vi "GetMethodImage.vi"(8 "error in (no error)":errorcluster, 9 "MethodVI":path, 10 "MethodName":string) -> (0 "error out":errorcluster, 2 "MethodImage":T2)   [LabVIEW 2020, in "ClassWriterNative.lvclass"]
uses:
  ClassWriterNative.lvclass
  <vilib>/picture/picture.llb/imagedata.ctl
  <vilib>/Utility/config.llb/Read Key (String).vi
  <vilib>/regexp/Match Regular Expression.xnode
  ClassWriterNative.lvclass/ClassWriterNative.ctl
  <vilib>/Utility/config.llb/NI_LVConfig.lvlib
panel:
  out "2D Picture":picture
  out "Array":T1(array[cluster])
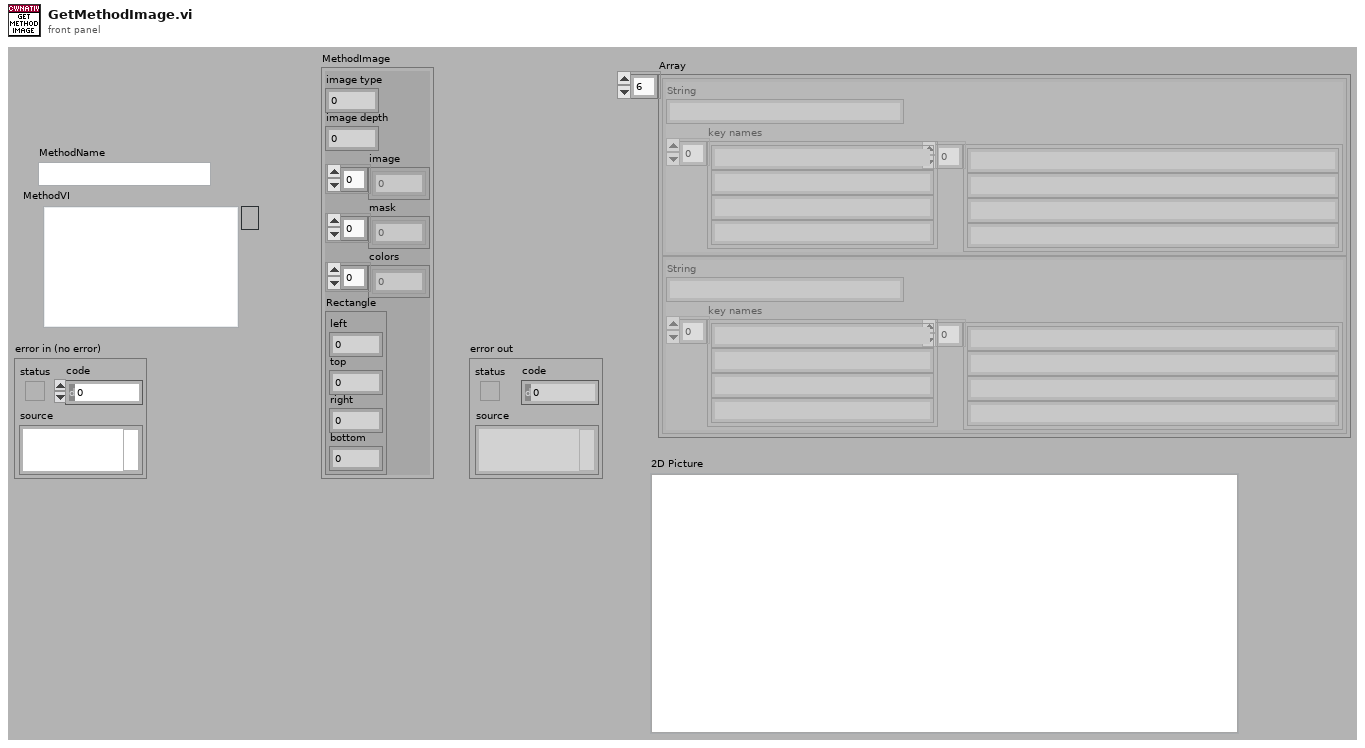
[diagram p1: front panel]
types:
  T1 = cluster{"String":string, "key names":string[], string[]}[]
  T2 = typedef "imagedata.ctl" = cluster{"image type":i32, "image depth":i32, "image":u8[], "mask":u8[], "colors":u32[], "Rectangle":cluster{"left":i16, "top":i16, "right":i16, "bottom":i16}}
  T3 = cluster{string, "key names":string[], string[]}[]
  T4 = typedef "NI_LVConfig.lvlib/Config Data RefNum.ctl" = refnum<k1>
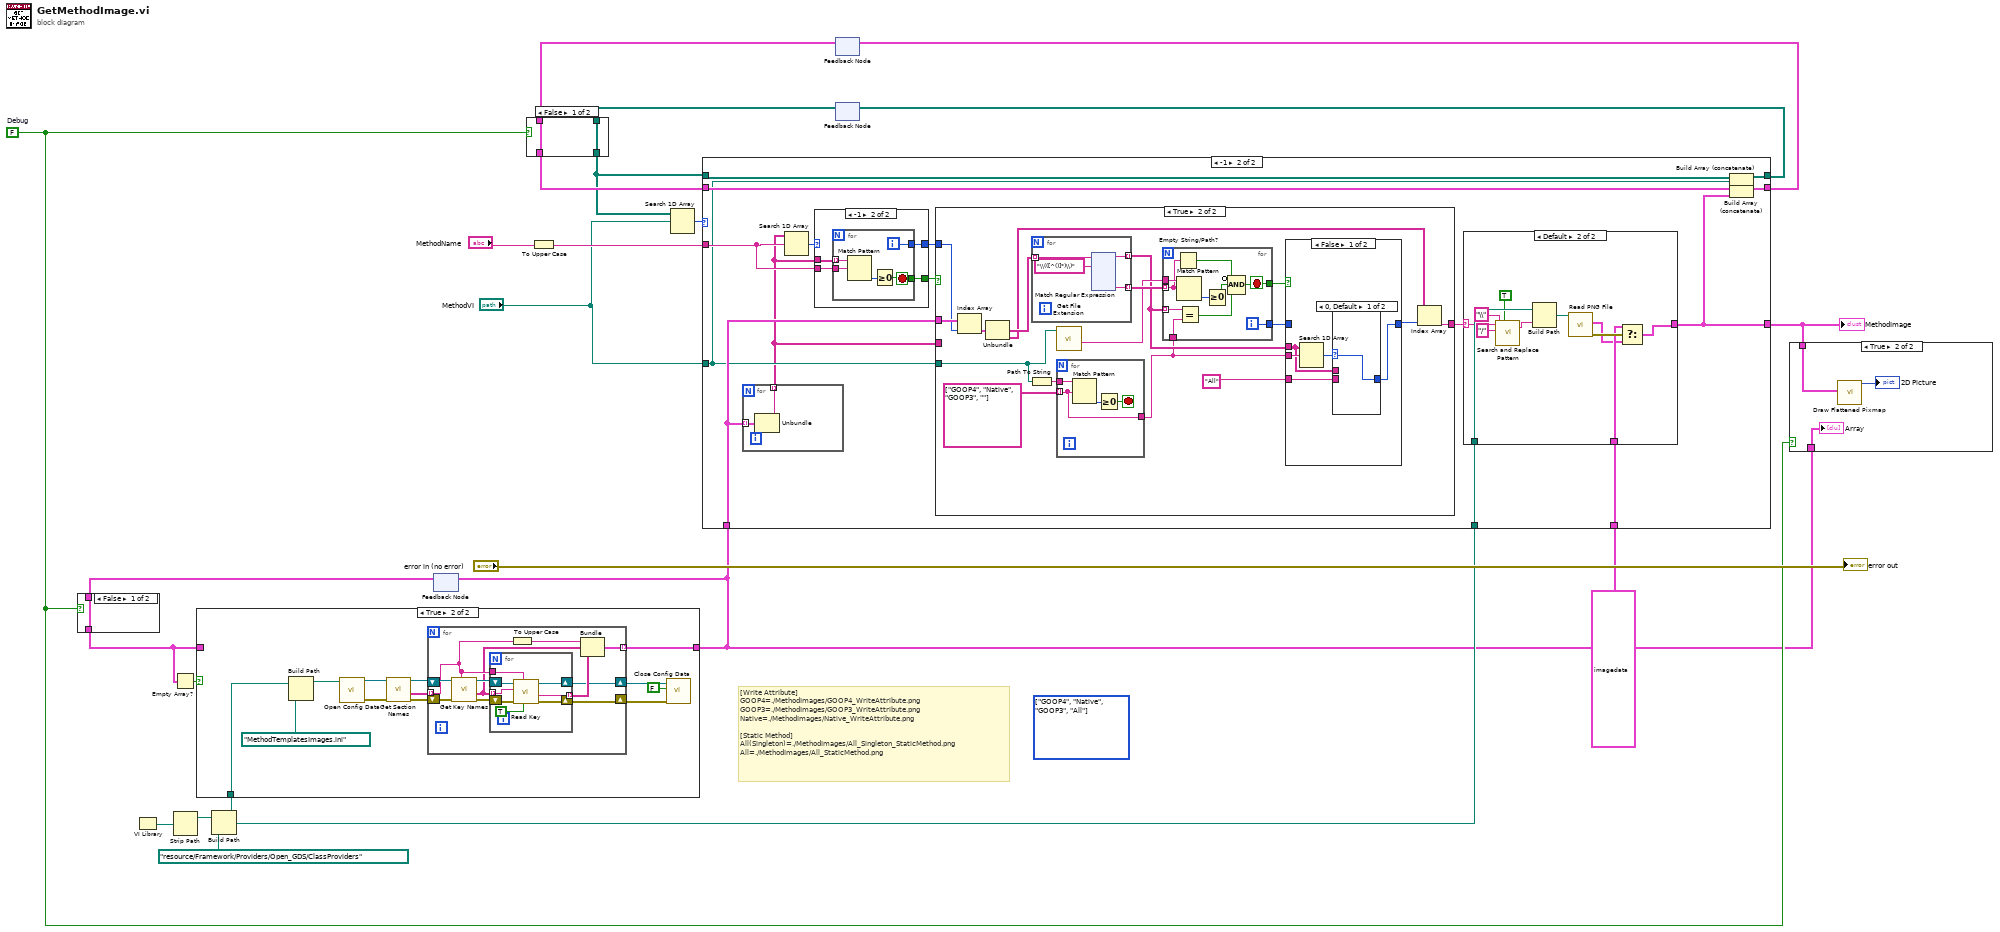
[diagram p0: block diagram]
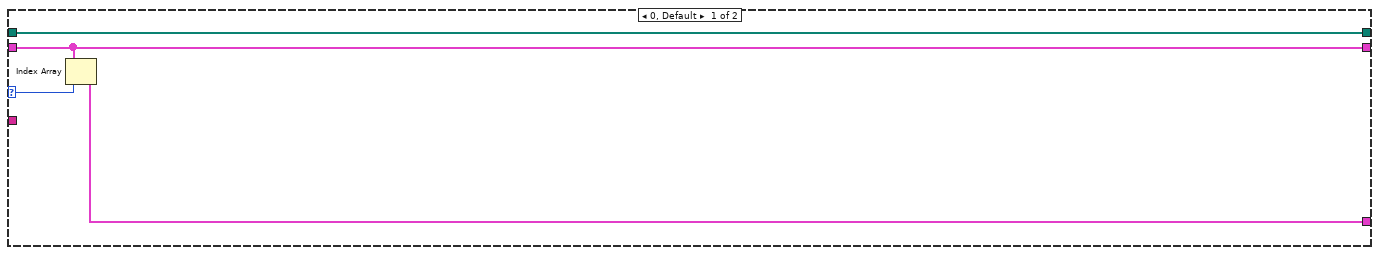
[diagram p6: hidden frame]
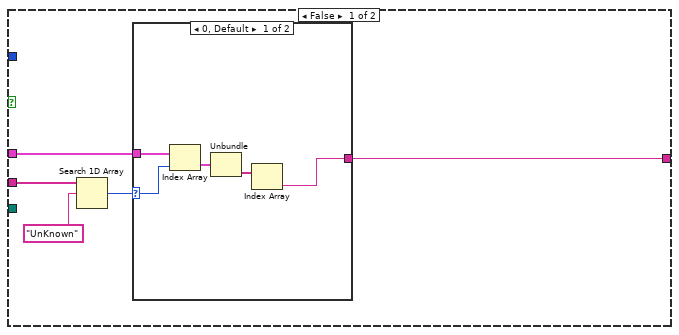
[diagram p8: hidden frame]
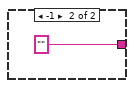
[diagram p9: hidden frame]
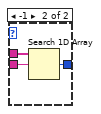
[diagram p10: hidden frame]
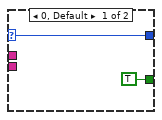
[diagram p12: hidden frame]
diagram:
  w3 = FALSE  # Debug
  (unwired) enum16{"Native", "GOOP3", "GOOP4", "All"}[] [enum."GOOP4", enum."Native", enum."GOOP3", enum."All"] items=["Native", "GOOP3", "GOOP4", "All"]
  # "[Write Attribute]\nGOOP4=./MethodImages/GOOP4_WriteAttribute.png\nGOOP3=./MethodImages/GOOP3_WriteAttribute.png\nNative=./MethodImages/Native_WriteAttribute.png\n\n[Static Method]\nAll(Singleton)=./MethodImages/All_Singleton_StaticMethod.png\nAll=./MethodImages/All_StaticMethod.png"
  n1 = VI Library() -> (path=w14:path)
  n2 = Strip Path(path=w14) -> (stripped path=w15:path)  [unwired: 1 out]
  n3 = Build Path(base path=w15, name or relative path=path "resource/Framework/Providers/Open_GDS/ClassProviders") -> (appended path=w12:path)
  n4 = feedback #1() -> (w7:T3)  [unwired: 1 in]
  n5 = case shown="False" w3 {
    tunnel: w7 -> [w23 _]
    tunnel: [w23 _] -> w6
    frame False {
    }
    frame True {
    }
  }
  n6 = Empty Array?(array=w6) -> (empty?=w16:bool)
  n7 = case shown="True" w16 {
    tunnel: [w24 w27] -> w2
    tunnel: w6 -> [w24 _]
    tunnel: w12 -> [_ w25]
    frame False {
    }
    frame True {
      n8 = Build Path(base path=w25, name or relative path=path "MethodTemplatesImages.ini") -> (appended path=w36:path)
      n9 = call <vilib>:"Open Config Data.vi"("configuration file path"=w36) -> ("error out"=w35:errorcluster, "refnum"=w34:T4)  [unwired: 8 in, 1 out]
      n10 = call <vilib>:"Get Section Names.vi"("error in (no error)"=w35, "refnum"=w34) -> ("error out"=w31:errorcluster, "section names"=w33:string[], "refnum out"=w32:T4)  [unwired: 7 in]
      n11 = for {
        tunnel: w33 -> [w44] mode=indexing
        shift-right: [w41] -> w30
        shift-left: w32 -> [w47]
        shift-right: [w40] -> w29
        shift-left: w31 -> [w46]
        tunnel: [w38] -> w27 mode=indexing
        n12 = call <vilib>:"Get Key Names.vi"("section"=w44, "error in (no error)"=w46, "refnum"=w47) -> ("error out"=w39:errorcluster, "key names"=w43:string[], "refnum out"=w45:T4)  [unwired: 5 in, 1 out]
        n13 = for {
          tunnel: w43 -> [w54] mode=indexing
          tunnel: w44 -> [w53]
          tunnel: [w52] -> w42 mode=indexing
          shift-right: [w51] -> w41
          shift-left: w45 -> [w55]
          shift-right: [w50] -> w40
          shift-left: w39 -> [w49]
          n14 = call-poly <vilib>:"Read Key.vi"("read raw string? (F)"=TRUE, "section"=w53, "error in (no error)"=w49, "key"=w54, "refnum"=w55) -> ("error out"=w50:errorcluster, "value"=w52:string, "refnum out"=w51:T4)  [unwired: 3 in, 1 out]
        }
        n15 = To Upper Case(1:w44) -> (0:w37:string)
        n16 = Bundle(w37, "key names"=w43, w42) -> (w38:cluster{string, "key names":string[], string[]})  [unwired: 1 in]
      }
      n17 = call <vilib>:"Close Config Data.vi"("error in (no error)"=w29, "write file if changed (T)"=FALSE, "refnum"=w30) -> ()  [unwired: 7 in, 2 out]
    }
  }
  n18 = feedback-in #1(w2) -> ()
  n19 = To Upper Case(1:"MethodName") -> (0:w4:string)
  n20 = feedback #2() -> (w19:T2[])  [unwired: 1 in]
  n21 = feedback #3() -> (w20:path[])  [unwired: 1 in]
  n22 = case shown="False" w3 {
    tunnel: w20 -> [w56 _]
    tunnel: w19 -> [w57 _]
    tunnel: [w57 _] -> w9
    tunnel: [w56 _] -> w8
    frame False {
    }
    frame True {
    }
  }
  n23 = Search 1D Array(1D array=w8, element="MethodVI") -> (index of element=w21:i32)  [unwired: 1 in]
  n24 = case shown="-1" w21 {
    selector: w21 -> [w61 _]
    tunnel: [w60 w72] -> w10
    tunnel: w4 -> [_ w75]
    tunnel: w8 -> [w58 w76]
    tunnel: w9 -> [w59 w73]
    tunnel: [w59 w71] -> w18
    tunnel: [w58 w74] -> w17
    tunnel: w2 -> [_ w70]
    tunnel: w12 -> [_ w69]
    tunnel: T2 {"image type"=0, "image depth"=24, "image"=array[188136 elements], "mask"=[], "colors"=[], "Rectangle"={"left"=0, "top"=0, "right"=312, "bottom"=201}} ("image data") -> [_ w68]
    tunnel: "MethodVI" -> [_ w67]
    frame 0, Default {
      n25 = Index Array(array=w59, index=w61) -> (element=w60:T2)
    }
    frame -1 {
      n26 = for {
        tunnel: w70 -> [w273] mode=indexing
        tunnel: [w272] -> w64 mode=indexing
        n27 = Unbundle(w273) -> (w272:string)  [unwired: 2 out]
      }
      n28 = Search 1D Array(1D array=w64, element=w75) -> (index of element=w66:i32)  [unwired: 1 in]
      n29 = case shown="-1" w66 {
        selector: w66 -> [w262 _]
        tunnel: w64 -> [_ w266]
        tunnel: w75 -> [_ w265]
        tunnel: [w262 w264] -> w62
        tunnel: [TRUE w263] -> w65
        frame 0, Default {
        }
        frame -1 {
          n30 = for {
            tunnel: w266 -> [w271] mode=indexing
            tunnel: w265 -> [w270]
            tunnel: [w268] -> w264
            tunnel: [w267] -> w263
            i -> [w268]
            stop <- w267 stop-if-true
            n31 = Match Pattern(string=w271, regular expression=w270) -> (offset past match=w269:i32)  [unwired: 1 in, 3 out]
            n32 = Greater Or Equal To 0?(x=w269) -> (x >= 0?=w267:bool)
          }
        }
      }
      n33 = case shown="True" w65 {
        tunnel: [w93 w105] -> w63
        tunnel: w64 -> [w92 _]
        tunnel: w70 -> [w89 w116]
        tunnel: w62 -> [_ w115]
        tunnel: w67 -> [_ w109]
        frame False {
          n34 = Search 1D Array(1D array=w92, element="UnKnown") -> (index of element=w90:i32)  [unwired: 1 in]
          n35 = case shown="0, Default" w90 {
            selector: w90 -> [w97 _]
            tunnel: [w94 ""] -> w93
            tunnel: w89 -> [w98 _]
            frame 0, Default {
              n36 = Index Array(array=w98, index=w97) -> (element=w96:cluster{string, "key names":string[], string[]})
              n37 = Unbundle(w96) -> (w95:string[])  [unwired: 2 out]
              n38 = Index Array(array=w95) -> (element=w94:string)  [unwired: 1 in]
            }
            frame -1 {
            }
          }
        }
        frame True {
          n39 = Index Array(array=w116, index=w115) -> (element=w114:cluster{string, "key names":string[], string[]})
          n40 = Unbundle(w114) -> ("key names"=w111:string[], w103:string[])  [unwired: 1 out]
          n41 = Path To String(path=w109) -> (string=w113:string)
          n42 = for {
            tunnel: w111 -> [w140] mode=indexing
            tunnel: [w138] -> w101 mode=indexing
            tunnel: [w137] -> w110 mode=indexing
            n43 = xnode "Match Regular Expression"("input string"=w140, "regular expression"="\\(([^()]*)\\)") -> ("before match"=w138:string, "submatch 1"=w137:string)  [unwired: 4 in, 4 out]
          }
          n44 = for {
            tunnel: w113 -> [w260]
            tunnel: string[] ["GOOP4", "Native", "GOOP3", ""] ("regular expression") -> [w257] mode=indexing
            tunnel: [w257] -> w100
            stop <- w258 stop-if-true
            n45 = Match Pattern(string=w260, regular expression=w257) -> (offset past match=w259:i32)  [unwired: 1 in, 3 out]
            n46 = Greater Or Equal To 0?(x=w259) -> (x >= 0?=w258:bool)
          }
          n47 = call <vilib>:"Get File Extension.vi"("file"=w109) -> ("filename without extension"=w108:string)  [unwired: 6 in, 4 out]
          n48 = for {
            tunnel: w110 -> [w135] mode=indexing
            tunnel: w108 -> [w136]
            tunnel: [w131] -> w107
            tunnel: [w130] -> w106
            tunnel: w101 -> [w129] mode=indexing
            tunnel: w100 -> [w128]
            i -> [w130]
            stop <- w131 stop-if-true
            n49 = Empty String/Path?(string/path=w135) -> (empty?=w134:bool)
            n50 = Match Pattern(string=w136, regular expression=w135) -> (offset past match=w133:i32)  [unwired: 1 in, 3 out]
            n51 = Equal?(x=w129, y=w128) -> (x = y?=w127:bool)
            n52 = Greater Or Equal To 0?(x=w133) -> (x >= 0?=w132:bool)
            n53 = Compound Arithmetic op=AND(invert w134, w132, w127) -> (w131:bool)
          }
          n54 = case shown="False" w107 {
            tunnel: w101 -> [w119 _]
            tunnel: w100 -> [w121 _]
            tunnel: w106 -> [_ w126]
            tunnel: [w117 w126] -> w104
            tunnel: "All" ("regular expression") -> [w118 _]
            frame False {
              n55 = Search 1D Array(1D array=w119, element=w121) -> (index of element=w120:i32)  [unwired: 1 in]
              n56 = case shown="0, Default" w120 {
                selector: w120 -> [w122 _]
                tunnel: w119 -> [_ w125]
                tunnel: w118 -> [_ w124]
                tunnel: [w122 w123] -> w117
                frame 0, Default {
                }
                frame -1 {
                  n57 = Search 1D Array(1D array=w125, element=w124) -> (index of element=w123:i32)  [unwired: 1 in]
                }
              }
            }
            frame True {
            }
          }
          n58 = Index Array(array=w103, index=w104) -> (element=w105:string)
        }
      }
      n59 = case shown="Default" w63 {
        selector: w63 -> [_ w82]
        tunnel: w69 -> [_ w88]
        tunnel: [w77 w83] -> w72
        tunnel: w68 -> [w77 w85]
        frame "" {
        }
        frame Default {
          n60 = call <vilib>:"Search and Replace Pattern.vi"("string"=w82, "regular expression (\"\")"="/" ("regular expression (\"\")"), "replace string (\"\")"="\\" ("replace string (\"\")"), "replace all? (F)"=TRUE) -> ("result string"=w81:string)  [unwired: 1 in, 1 out]
          n61 = Build Path(base path=w88, name or relative path=w81) -> (appended path=w87:path)
          n62 = call <vilib>:"Read PNG File.vi"("path to PNG file"=w87) -> ("error out"=w86:errorcluster, "image data"=w84:T2)  [unwired: 8 in, 1 out]
          n63 = Select(t=w85, s=w86, f=w84) -> (s? t:f=w83:T2)
        }
      }
      n64 = Build Array (concatenate)(w76, w67) -> (w74:path[])
      n65 = Build Array (concatenate)(w73, w72) -> (w71:T2[])
    }
  }
  "MethodImage" <- w10
  n66 = feedback-in #2(w18) -> ()
  n67 = feedback-in #3(w17) -> ()
  n68 = case shown="True" w3 {
    tunnel: w10 -> [_ w276]
    tunnel: w2 -> [_ w274]
    frame False {
    }
    frame True {
      n69 = call <vilib>:"Draw Flattened Pixmap.vi"("image data"=w276) -> ("new picture"=→"2D Picture":picture)  [unwired: 8 in]
      "Array" <- w274
    }
  }
  "error out" <- "error in (no error)"
